vi "CalcCalibrGraph (SubVI).vi"(10 "K":dbl, 11 "TableMeasAmpl":string[][](array[string])) -> (2 "Array 2":dbl[][](array[numeric]), 3 "Array":cluster{dbl[], dbl[]}[](array[cluster]))   [LabVIEW 2017]
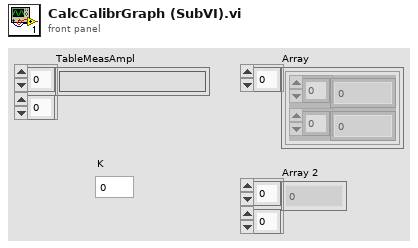
[diagram p1: front panel]
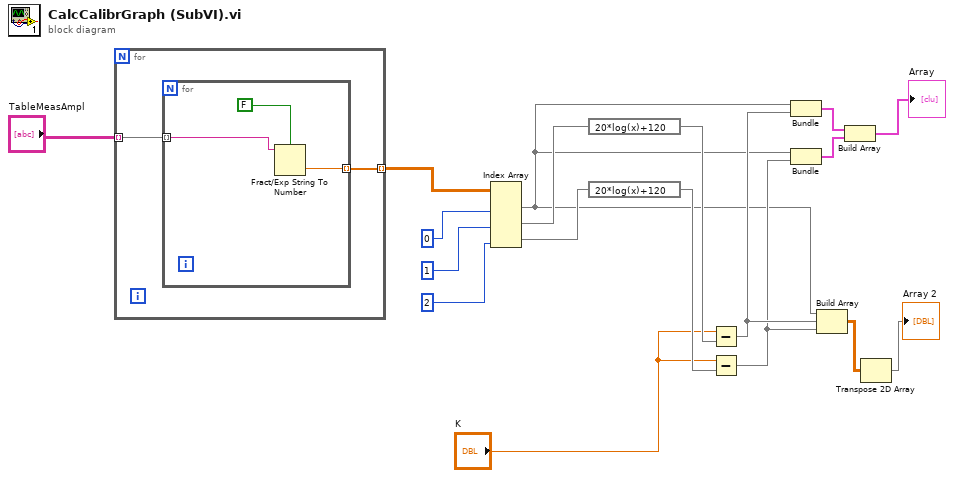
[diagram p0: block diagram]
diagram:
  n1 = for {
    tunnel: "TableMeasAmpl" -> [w20] mode=indexing
    tunnel: [w19] -> w14 mode=indexing
    n2 = for {
      tunnel: w20 -> [w23] mode=indexing
      tunnel: [w22] -> w19 mode=indexing
      n3 = Fract/Exp String To Number(use system decimal point (T)=FALSE, string=w23) -> (number=w22:dbl)  [unwired: 2 in, 1 out]
    }
  }
  n4 = Index Array(array=w14, index (col) #1=0 ("disabled index (col)"), index (col) #2=1 ("index (col)"), index (col) #3=2 ("index (col)")) -> (element #1=w1:dbl[], element #2=w10:dbl[], element #3=w9:dbl[])  [unwired: 3 in]
  n5 = expression code="20*log(x)+120"(w10) -> (w8:dbl[])
  n6 = expression code="20*log(x)+120"(w9) -> (w7:dbl[])
  n7 = Subtract(x="K", y=w8) -> (x-y=w5:dbl[])
  n8 = Subtract(x="K", y=w7) -> (x-y=w4:dbl[])
  n9 = Bundle(w1, w5) -> (w13:cluster{dbl[], dbl[]})  [unwired: 1 in]
  n10 = Bundle(w1, w4) -> (w12:cluster{dbl[], dbl[]})  [unwired: 1 in]
  n11 = Build Array(w1, w5, w4) -> (w3:dbl[][])
  n12 = Build Array(w13, w12) -> (→"Array":cluster{dbl[], dbl[]}[])
  n13 = Transpose 2D Array(2D array=w3) -> (transposed array=→"Array 2":dbl[][])
